vi "Unpack welcome byte.vi"(11 "Byte":u8[](array[numeric]) format="%x") -> (0 "error (out)":errorcluster, 3 "Length (octets)":u8 format="%b")   [LabVIEW 2020, in "wamplv.lvlib" / "RawSocket TCP Handler.lvclass"]
uses:
  RawSocket TCP Handler.lvclass
  <vilib>/Utility/error.llb/Error Cluster From Error Code.vi
  <vilib>/ErrorRing/Error Ring.xnode
  RawSocket TCP Handler.lvclass/RawSocket TCP Handler.ctl
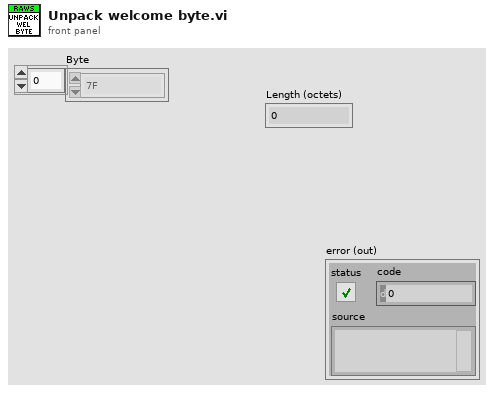
[diagram p1: front panel]
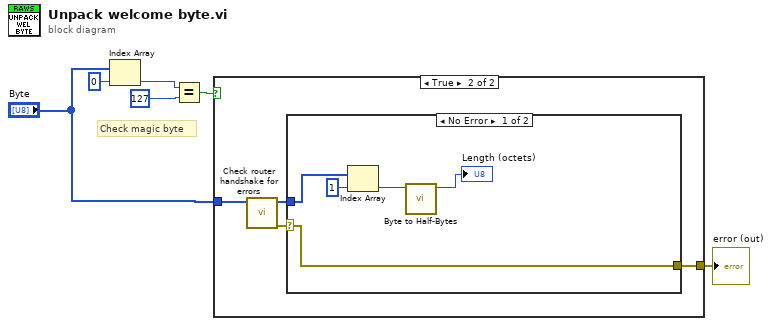
[diagram p0: block diagram]
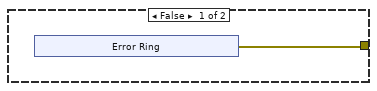
[diagram p2: hidden frame]
diagram:
  # "Check magic byte"
  n1 = Index Array(array="Byte", index=0) -> (element=w4:u8)
  n2 = Equal?(x=w4, y=u8 127) -> (x = y?=w3:bool)
  n3 = case shown="True" w3 {
    tunnel: "Byte" -> [_ w15]
    tunnel: [w7 w12] -> w1
    frame False {
      n4 = xnode "Error Ring"() -> ("error out"=w7:errorcluster)
    }
    frame True {
      n5 = call "Check router handshake for errors.vi"("Bytes (in)"=w15) -> ("error out"=w14:errorcluster, "Byte (out)"=w13:u8[])  [unwired: 9 in]
      n6 = case shown="No Error" w14 {
        selector: w14 -> [w17 w21]
        tunnel: w13 -> [w20 _]
        tunnel: [w17 w21] -> w12
        frame No Error {
          n7 = Index Array(array=w20, index=1) -> (element=w18:u8)
          n8 = call "Byte to Half-Bytes.vi"("Byte In"=w18) -> ("Upper Half-Byte"=→"Length (octets)":u8)  [unwired: 7 in, 1 out]
        }
        frame Error {
        }
      }
    }
  }
  "error (out)" <- w1
